vi "CmdControl _ch_1-20.vi"() -> (1 "Dataout":u8[](array[numeric]))   [LabVIEW 2017]
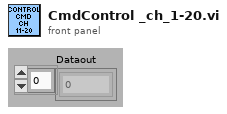
[diagram p1: front panel]
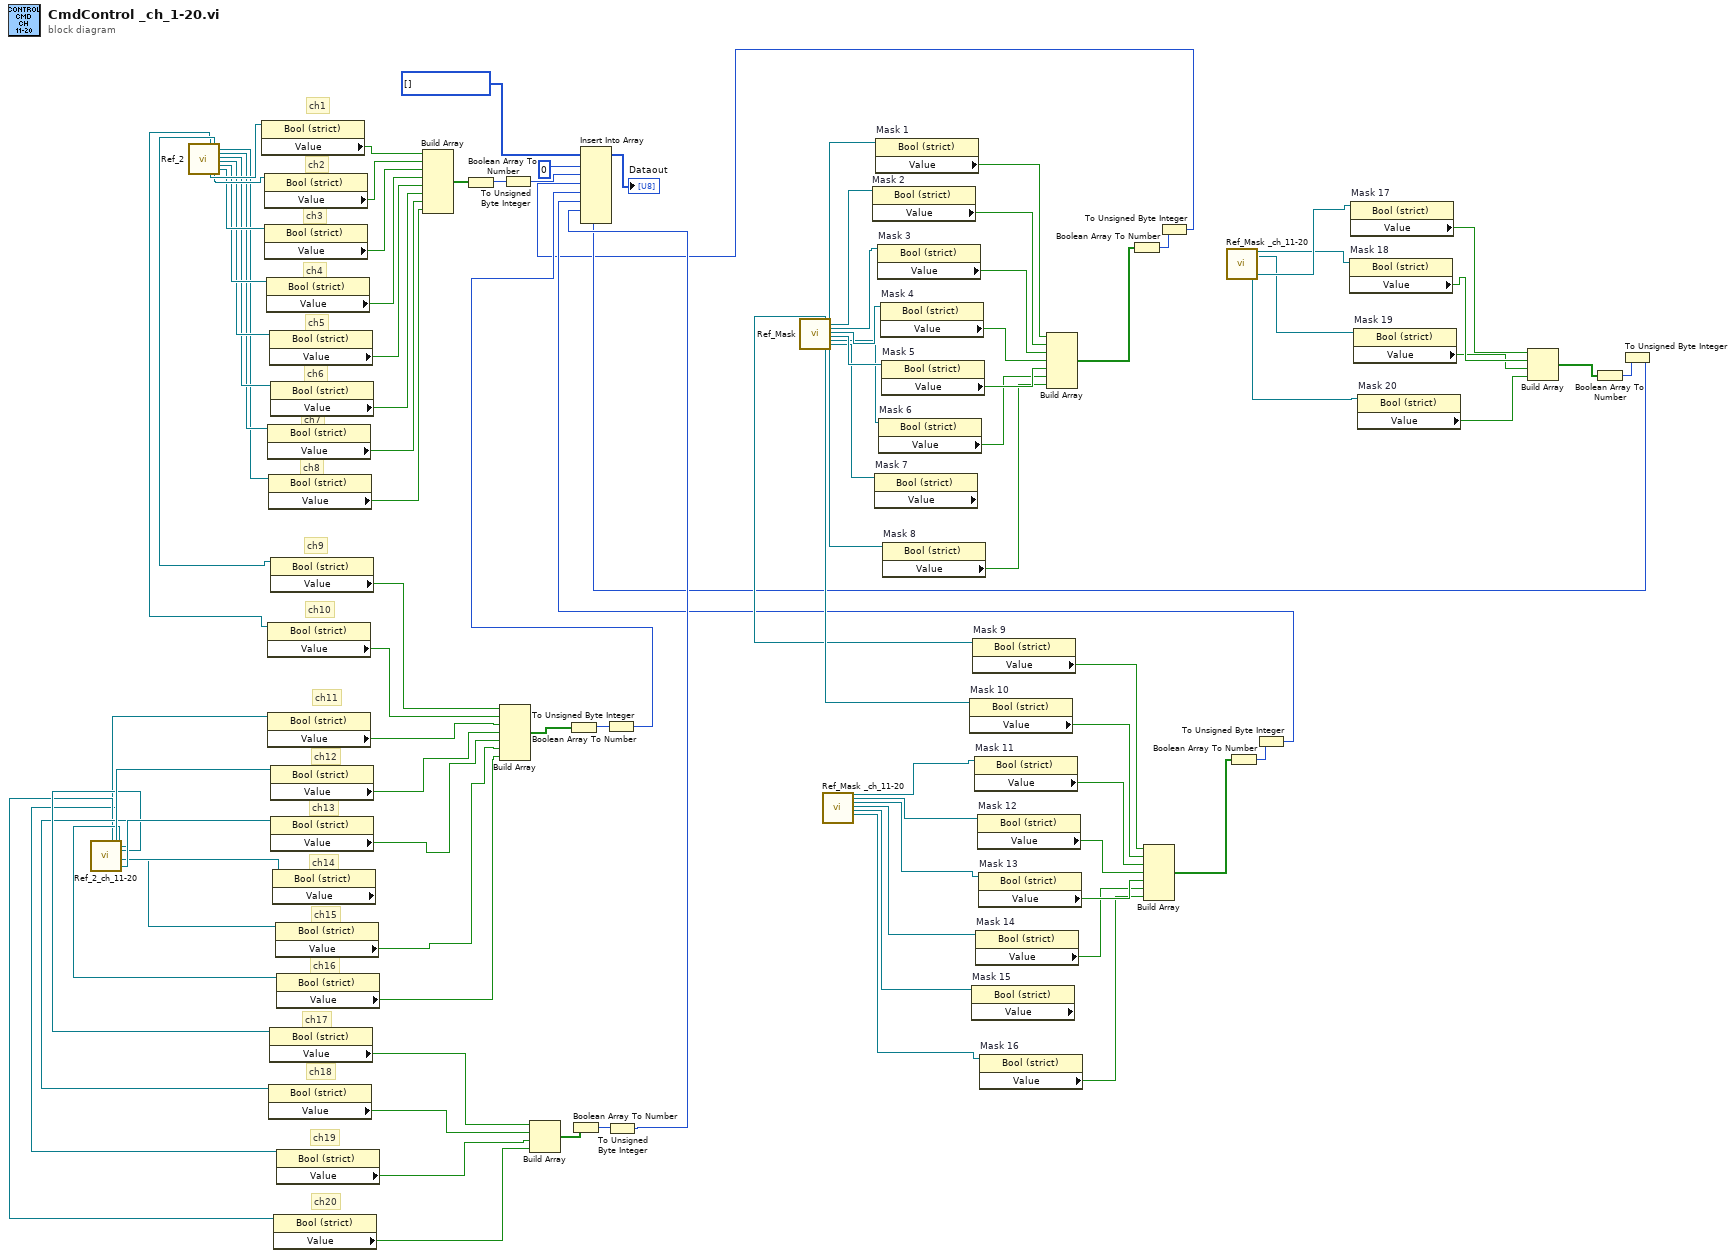
[diagram p0: block diagram]
diagram:
  # "ch20"
  # "ch19"
  # "ch18"
  # "ch17"
  # "ch16"
  # "ch15"
  # "ch14"
  # "ch13"
  # "ch12"
  # "ch11"
  # "ch10"
  # "ch9"
  # "ch8"
  # "ch7"
  # "ch6"
  # "ch5"
  # "ch4"
  # "ch3"
  # "ch2"
  # "ch1"
  n1 = call "Ref_2_ch_11-20.vi"() -> ("Control  Ch 20 out"=w67:refnum<vi>, "Control  Ch 11 out"=w66:refnum<vi>, "Control  Ch 19 out"=w65:refnum<vi>, "Control  Ch 12 out"=w74:refnum<vi>, "Control  Ch 18 out"=w68:refnum<vi>, "Control  Ch 17 out"=w69:refnum<vi>, "Control  Ch 16 out"=w70:refnum<vi>, "Control  Ch 15 out"=w71:refnum<vi>, "Control  Ch 14 out"=w72:refnum<vi>, "Control  Ch 13 out"=w73:refnum<vi>)  [unwired: 17 in, 1 out]
  n2 = call "Ref_2.vi"() -> ("Control  Ch 10 out"=w75:refnum<vi>, "Control  Ch 1 out"=w96:refnum<vi>, "Control  Ch 9 out"=w76:refnum<vi>, "Control  Ch 2 out"=w95:refnum<vi>, "Control  Ch 8 out"=w89:refnum<vi>, "Control  Ch 7 out"=w90:refnum<vi>, "Control  Ch 6 out"=w91:refnum<vi>, "Control  Ch 5 out"=w92:refnum<vi>, "Control  Ch 4 out"=w93:refnum<vi>, "Control  Ch 3 out"=w94:refnum<vi>)  [unwired: 17 in, 1 out]
  n3 = property class="Bool (strict)"(reference=w96) -> ("Value"=w88:bool)  [unwired: 1 in, 2 out]
  n4 = property class="Bool (strict)"(reference=w95) -> ("Value"=w87:bool)  [unwired: 1 in, 2 out]
  n5 = property class="Bool (strict)"(reference=w94) -> ("Value"=w86:bool)  [unwired: 1 in, 2 out]
  n6 = property class="Bool (strict)"(reference=w93) -> ("Value"=w85:bool)  [unwired: 1 in, 2 out]
  n7 = property class="Bool (strict)"(reference=w90) -> ("Value"=w82:bool)  [unwired: 1 in, 2 out]
  n8 = property class="Bool (strict)"(reference=w75) -> ("Value"=w63:bool)  [unwired: 1 in, 2 out]
  n9 = property class="Bool (strict)"(reference=w66) -> ("Value"=w62:bool)  [unwired: 1 in, 2 out]
  n10 = property class="Bool (strict)"(reference=w89) -> ("Value"=w81:bool)  [unwired: 1 in, 2 out]
  n11 = property class="Bool (strict)"(reference=w68) -> ("Value"=w52:bool)  [unwired: 1 in, 2 out]
  n12 = property class="Bool (strict)"(reference=w92) -> ("Value"=w84:bool)  [unwired: 1 in, 2 out]
  n13 = property class="Bool (strict)"(reference=w69) -> ("Value"=w53:bool)  [unwired: 1 in, 2 out]
  n14 = property class="Bool (strict)"(reference=w91) -> ("Value"=w83:bool)  [unwired: 1 in, 2 out]
  n15 = property class="Bool (strict)"(reference=w76) -> ("Value"=w64:bool)  [unwired: 1 in, 2 out]
  n16 = property class="Bool (strict)"(reference=w74) -> ("Value"=w61:bool)  [unwired: 1 in, 2 out]
  n17 = property class="Bool (strict)"(reference=w73) -> ("Value"=w60:bool)  [unwired: 1 in, 2 out]
  n18 = property class="Bool (strict)" props=["Value"](reference=w72) -> ()  [unwired: 1 in, 3 out]
  n19 = property class="Bool (strict)"(reference=w67) -> ("Value"=w50:bool)  [unwired: 1 in, 2 out]
  n20 = property class="Bool (strict)"(reference=w71) -> ("Value"=w59:bool)  [unwired: 1 in, 2 out]
  n21 = property class="Bool (strict)"(reference=w70) -> ("Value"=w58:bool)  [unwired: 1 in, 2 out]
  n22 = property class="Bool (strict)"(reference=w65) -> ("Value"=w51:bool)  [unwired: 1 in, 2 out]
  n23 = Build Array(w88, w87, w86, w85, w84, w83, w82, w81) -> (w80:bool[])
  n24 = Boolean Array To Number(Boolean array=w80) -> (number=w79:u32)
  n25 = Build Array(w64, w63, w62, w61, w60, w59, w58) -> (w56:bool[])
  n26 = To Unsigned Byte Integer(number=w79) -> (unsigned 8bit integer=w78:u8)
  n27 = Build Array(w53, w52, w51, w50) -> (w54:bool[])
  n28 = Boolean Array To Number(Boolean array=w56) -> (number=w57:u32)
  n29 = Boolean Array To Number(Boolean array=w54) -> (number=w48:u32)
  n30 = To Unsigned Byte Integer(number=w57) -> (unsigned 8bit integer=w55:u8)
  n31 = To Unsigned Byte Integer(number=w48) -> (unsigned 8bit integer=w49:u8)
  n32 = call "Ref_Mask.vi"() -> ("Mask Ch 9 out"=w20:refnum<vi>, "Mask Ch 10 out"=w21:refnum<vi>, "Mask Ch 1 out"=w39:refnum<vi>, "Mask Ch 2 out"=w38:refnum<vi>, "Mask Ch 3 out"=w37:refnum<vi>, "Mask Ch 4 out"=w36:refnum<vi>, "Mask Ch 5 out"=w35:refnum<vi>, "Mask Ch 6 out"=w34:refnum<vi>, "Mask Ch 7 out"=w33:refnum<vi>, "Mask Ch 8 out"=w32:refnum<vi>)  [unwired: 18 in]
  n33 = call "Ref_Mask _ch_11-20.vi"() -> ("Mask Ch 11 out"=w19:refnum<vi>, "Mask Ch 12 out"=w18:refnum<vi>, "Mask Ch 13 out"=w17:refnum<vi>, "Mask Ch 14 out"=w16:refnum<vi>, "Mask Ch 15 out"=w15:refnum<vi>, "Mask Ch 16 out"=w14:refnum<vi>)  [unwired: 18 in, 4 out]
  n34 = property on="Mask 2" class="Bool (strict)"(reference=w38) -> ("Value"=w44:bool)  [unwired: 1 in, 2 out]
  n35 = property on="Mask 7" class="Bool (strict)" props=["Value"](reference=w33) -> ()  [unwired: 1 in, 3 out]
  n36 = property on="Mask 1" class="Bool (strict)"(reference=w39) -> ("Value"=w45:bool)  [unwired: 1 in, 2 out]
  n37 = property on="Mask 3" class="Bool (strict)"(reference=w37) -> ("Value"=w43:bool)  [unwired: 1 in, 2 out]
  n38 = property on="Mask 6" class="Bool (strict)"(reference=w34) -> ("Value"=w40:bool)  [unwired: 1 in, 2 out]
  n39 = property on="Mask 4" class="Bool (strict)"(reference=w36) -> ("Value"=w42:bool)  [unwired: 1 in, 2 out]
  n40 = property on="Mask 5" class="Bool (strict)"(reference=w35) -> ("Value"=w41:bool)  [unwired: 1 in, 2 out]
  n41 = property on="Mask 8" class="Bool (strict)"(reference=w32) -> ("Value"=w31:bool)  [unwired: 1 in, 2 out]
  n42 = property on="Mask 10" class="Bool (strict)"(reference=w21) -> ("Value"=w27:bool)  [unwired: 1 in, 2 out]
  n43 = property on="Mask 15" class="Bool (strict)" props=["Value"](reference=w15) -> ()  [unwired: 1 in, 3 out]
  n44 = property on="Mask 9" class="Bool (strict)"(reference=w20) -> ("Value"=w28:bool)  [unwired: 1 in, 2 out]
  n45 = property on="Mask 11" class="Bool (strict)"(reference=w19) -> ("Value"=w26:bool)  [unwired: 1 in, 2 out]
  n46 = property on="Mask 14" class="Bool (strict)"(reference=w16) -> ("Value"=w23:bool)  [unwired: 1 in, 2 out]
  n47 = property on="Mask 12" class="Bool (strict)"(reference=w18) -> ("Value"=w25:bool)  [unwired: 1 in, 2 out]
  n48 = property on="Mask 13" class="Bool (strict)"(reference=w17) -> ("Value"=w24:bool)  [unwired: 1 in, 2 out]
  n49 = property on="Mask 16" class="Bool (strict)"(reference=w14) -> ("Value"=w22:bool)  [unwired: 1 in, 2 out]
  n50 = Build Array(w45, w44, w43, w42, w41, w40, w31) -> (w46:bool[])
  n51 = Boolean Array To Number(Boolean array=w46) -> (number=w47:u32)
  n52 = Build Array(w28, w27, w26, w25, w24, w23, w22) -> (w29:bool[])
  n53 = To Unsigned Byte Integer(number=w47) -> (unsigned 8bit integer=w1:u8)
  n54 = call "Ref_Mask _ch_11-20.vi"() -> ("Mask Ch 19 out"=w10:refnum<vi>, "Mask Ch 20 out"=w11:refnum<vi>, "Mask Ch 17 out"=w13:refnum<vi>, "Mask Ch 18 out"=w12:refnum<vi>)  [unwired: 18 in, 6 out]
  n55 = Boolean Array To Number(Boolean array=w29) -> (number=w30:u32)
  n56 = To Unsigned Byte Integer(number=w30) -> (unsigned 8bit integer=w2:u8)
  n57 = property on="Mask 18" class="Bool (strict)"(reference=w12) -> ("Value"=w6:bool)  [unwired: 1 in, 2 out]
  n58 = property on="Mask 17" class="Bool (strict)"(reference=w13) -> ("Value"=w7:bool)  [unwired: 1 in, 2 out]
  n59 = property on="Mask 19" class="Bool (strict)"(reference=w10) -> ("Value"=w5:bool)  [unwired: 1 in, 2 out]
  n60 = property on="Mask 20" class="Bool (strict)"(reference=w11) -> ("Value"=w4:bool)  [unwired: 1 in, 2 out]
  n61 = Build Array(w7, w6, w5, w4) -> (w8:bool[])
  n62 = Boolean Array To Number(Boolean array=w8) -> (number=w9:u32)
  n63 = To Unsigned Byte Integer(number=w9) -> (unsigned 8bit integer=w3:u8)
  n64 = Insert Into Array(array=u8[] [] ("Data 2"), index=0, new element #1=w78, new element #2=w1, new element #3=w55, new element #4=w2, new element #5=w49, new element #6=w3) -> (→"Dataout":u8[])
